vi "Dequeue Element.vi"(8 "error in (no error)":errorcluster, 9 "Timeout In ms (-1)":i32=-1, 11 "Priority Queue":T1) -> (0 "error out":errorcluster, 1 "Timed Out?":bool, 2 "Cross JKI State Machine State":T2, 3 "Priority Queue (Dup)":T1, 4 "High Priority?":bool)   [LabVIEW 2017, in "Communicable State Machine.lvlib"]
doc: "### Dequeue Element.vi\n\n-- <b>Controls</b> --\n- <b>timeout in ms (-1)</b>:\n- <b>Priority Queue</b>:\n\n-- <b>Indicators</b> --\n- <b>timed out?</b>:\n- <b>Cross JKI State Machine State</b>:\n- <b>Priority Queue(dup)</b>:\n- <b>High Priority?</b>:"
uses:
  Communicable State Machine.lvlib
  Priority Queue.ctl
  Typedef/_Cross CSM State Data.ctl
  Typedef/_CSM_MSG_TYPE.ctl
  Typedef/_Cross CSM State Response.ctl
  Typedef/_CSM_Response Source Message.ctl
  def-Data(LowPRI-Q).ctl
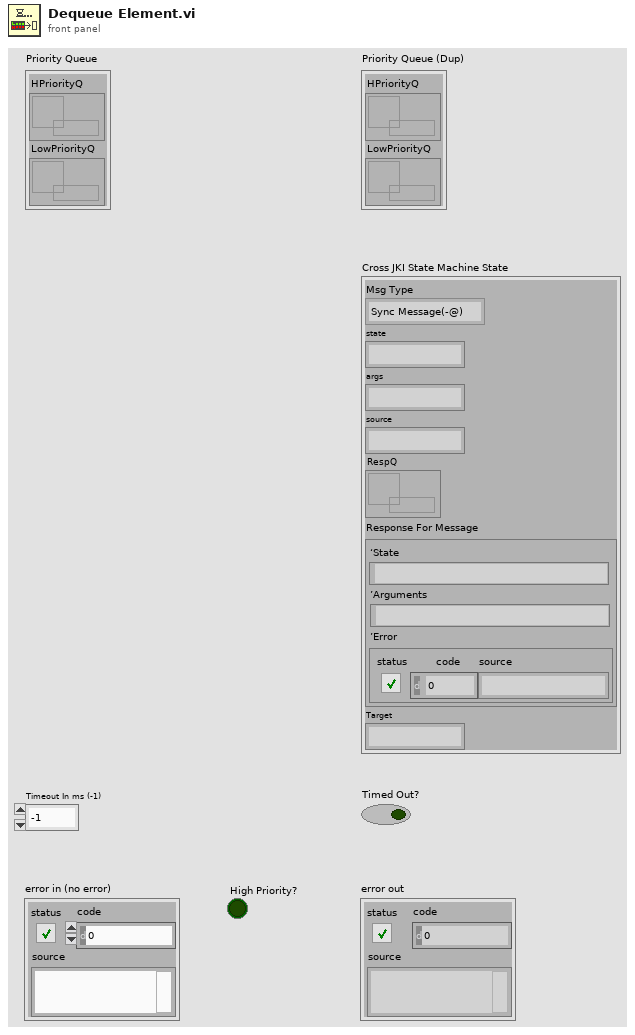
[diagram p1: front panel]
types:
  T1 = typedef "Communicable State Machine.lvlib/Priority Queue.ctl" = cluster{"HPriorityQ":refnum<queue>, "LowPriorityQ":refnum<queue>}
  T2 = typedef "Communicable State Machine.lvlib/_Cross CSM State Data.ctl" = cluster{"Msg Type":T3, "state":string, "args":string, "source":string, "RespQ":refnum<queue>, "Response For Message":T4, "Target":string}
  T3 = typedef "Communicable State Machine.lvlib/_CSM_MSG_TYPE.ctl" = enum16{"Sync Message(-@)", "Async Message(->)", "Async without Response(->|)", "Async Response", "Broadcast(-><all>)", "Broadcast(-><status>)", "Broadcast(-><interrupt>)", "Append to JKISM States", "Append to JKISM States(High Priority)", "Broadcast(-><state>)"}
  T4 = typedef "Communicable State Machine.lvlib/_CSM_Response Source Message.ctl" = cluster{"‘State":string, "’Arguments":string, "’Error":errorcluster}
  T5 = typedef "Communicable State Machine.lvlib/def-Data(LowPRI-Q).ctl" = cluster{"Data":T2, "Notify?":bool}
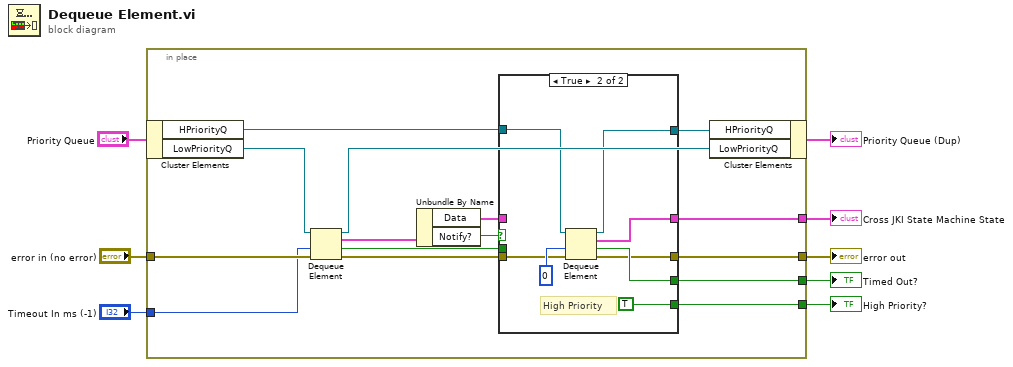
[diagram p0: block diagram]
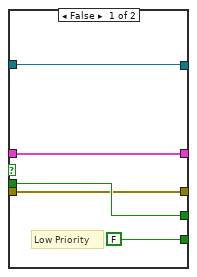
[diagram p2: hidden frame]
diagram:
  n1 = in-place {
    in-place-border: [w23] -> w8
    in-place-border: "error in (no error)" -> [w22]
    in-place-border: [w21] -> w6
    in-place-border: [w20] -> w5
    in-place-border: [w19] -> w4
    in-place-border: "Timeout In ms (-1)" -> [w18]
    n2 = in-place-cluster #1("Priority Queue") -> ("HPriorityQ"=w12:refnum<queue>, "LowPriorityQ"=w11:refnum<queue>)
    n3 = Dequeue Element(queue=w11, timeout in ms (-1)=w18, error in (no error)=w22) -> (queue out=w10:refnum<queue>, element=w17:T5, timed out?=w14:bool, error out=w13:errorcluster)
    n4 = Unbundle By Name(w17) -> ("Data"=w15:T2, "Notify?"=w16:bool)
    n5 = case shown="True" w16 {
      tunnel: w12 -> [w24 w36]
      tunnel: w15 -> [w28 _]
      tunnel: [w28 w34] -> w19
      tunnel: [FALSE TRUE] -> w20
      tunnel: [w26 w32] -> w21
      tunnel: w14 -> [w26 _]
      tunnel: w13 -> [w25 w31]
      tunnel: [w25 w30] -> w23
      tunnel: [w24 w29] -> w9
      frame False {
        # "Low Priority"
      }
      frame True {
        # "High Priority"
        n6 = Dequeue Element(queue=w36, timeout in ms (-1)=0, error in (no error)=w31) -> (queue out=w29:refnum<queue>, element=w34:T2, timed out?=w32:bool, error out=w30:errorcluster)
      }
    }
    n7 = in-place-cluster #1("HPriorityQ"=w9, "LowPriorityQ"=w10) -> (→"Priority Queue (Dup)":T1)
  }
  "error out" <- w8
  "Timed Out?" <- w6
  "High Priority?" <- w5
  "Cross JKI State Machine State" <- w4
